vi "MyrioProject.vi"() -> ()   [LabVIEW 2018]
doc: "The myRIO Project template acquires acceleration data from the onboard accelerometer and displays the changes of acceleration values in a waveform chart."
uses:
  <vilib>/myRIO/Common/Instrument Driver Framework/myRIO v1.0/Encoder/typedefs/Encoder Signal Mode.ctl
  <vilib>/Platform/TimedLoop/XDataNode/timing_clust.ctl
  <vilib>/Platform/TimedLoop/XDataNode/nitl_modes.ctl
  <vilib>/Platform/TimedLoop/XDataNode/wakeup.ctl
  <vilib>/Analysis/Matrix/Datatypes/RealMatrix.ctl
  <vilib>/myRIO/Instrument Drivers/Onboard IO/PWM/typedefs/PWM Reference.ctl
  <vilib>/myRIO/Common/Instrument Driver Framework/Utilities/typedefs/myRIO Generic Hardware Reference.ctl
  <vilib>/myRIO/Common/Instrument Driver Framework/Utilities/typedefs/Hardware Version Enum.ctl
  <vilib>/myRIO/Common/Instrument Driver Framework/Utilities/typedefs/myRIO v1.0 Reference.ctl
  <vilib>/myRIO/Common/Instrument Driver Framework/Utilities/typedefs/Generic FPGA Reference.ctl
  <vilib>/myRIO/Common/Instrument Driver Framework/myRIO v1.0/PWM/typedefs/PWM Channels Enum.ctl
  <vilib>/myRIO/Instrument Drivers/Onboard IO/PWM/typedefs/PWM Configuration.ctl
  <vilib>/userdefined/High Color/nirio_resource_hc.ctl
  <vilib>/myRIO/Common/Instrument Driver Framework/myRIO v1.0/Encoder/typedefs/Encoder Configuration v1.0.ctl
  <vilib>/myRIO/Instrument Drivers/Onboard IO/Encoder/typedefs/Encoder Reference.ctl
  <vilib>/myRIO/Common/Instrument Driver Framework/myRIO v1.0/Encoder/typedefs/Encoder Channels Enum.ctl
  <vilib>/myRIO/Instrument Drivers/Onboard IO/DIO/typedefs/DIO Reference.ctl
  <vilib>/myRIO/Common/Instrument Driver Framework/myRIO v1.0/DIO/typedefs/DIO Channels List.ctl
  <vilib>/myRIO/Common/Instrument Driver Framework/myRIO v1.0/DIO/typedefs/DIO Channels Enum.ctl
  <vilib>/myRIO/Instrument Drivers/Onboard IO/AI/typedefs/AI Reference.ctl
  <vilib>/myRIO/Common/Instrument Driver Framework/myRIO v1.0/AI/typedefs/AI Channels List.ctl
  <vilib>/myRIO/Common/Instrument Driver Framework/myRIO v1.0/AI/typedefs/AI Channels Enum.ctl
  <vilib>/myRIO/Common/Instrument Driver Framework/Utilities/typedefs/Analog Scaling Constants List.ctl
  <vilib>/myRIO/Common/Instrument Driver Framework/Utilities/typedefs/Analog Scaling Constants.ctl
  <vilib>/myRIO/Common/Instrument Driver Framework/myRIO v1.0/PWM/vis/myRIO v1.1 Open PWM.vi
  <vilib>/myRIO/Common/Instrument Driver Framework/myRIO v1.0/Encoder/vis/myRIO v1.1 Open Encoder.vi
  <vilib>/myRIO/Common/Instrument Driver Framework/Utilities/vis/Is FPGA Ref Available.vi
  <vilib>/myRIO/Common/Instrument Driver Framework/myRIO v1.0/AI/vis/myRIO v1.1 Open AI.vi
  <vilib>/myRIO/Common/Instrument Driver Framework/myRIO v1.0/DIO/vis/myRIO v1.1 Open DIO.vi
  <vilib>/myRIO/Instrument Drivers/Onboard IO/PWM/vis/Set Duty Cycle and Frequency.vi
  <vilib>/myRIO/Instrument Drivers/Onboard IO/DIO/vis/Write.vi
  <vilib>/myRIO/Common/Instrument Driver Framework/Utilities/vis/Validate Channels.vi
  <vilib>/myRIO/Common/Instrument Driver Framework/myRIO v1.0/PWM/vis/myRIO v1.0 Reserve PWM.vi
  <vilib>/myRIO/Common/Instrument Driver Framework/myRIO v1.0/Encoder/vis/myRIO v1.0 Reserve Encoder.vi
  <vilib>/myRIO/Common/Instrument Driver Framework/myRIO v1.0/AI/vis/myRIO v1.0 Reserve AI.vi
  <vilib>/myRIO/Common/Instrument Driver Framework/myRIO v1.0/DIO/vis/myRIO v1.0 Reserve DIO.vi
  <vilib>/myRIO/Common/Instrument Driver Framework/myRIO v1.0/Encoder/vis/myRIO v1.0 Close Encoder.vi
  <vilib>/myRIO/Common/Instrument Driver Framework/myRIO v1.0/PWM/vis/myRIO v1.0 Close PWM.vi
  <vilib>/myRIO/Common/Instrument Driver Framework/myRIO v1.0/PWM/vis/myRIO v1.0 Build MUX Configuration PWM.vi
  <vilib>/myRIO/Common/Instrument Driver Framework/myRIO v1.0/Resource Manager/vis/myRIO v1.0 Reserve Channel List.vi
  <vilib>/myRIO/Common/Instrument Driver Framework/myRIO v1.0/Encoder/vis/myRIO v1.0 Build MUX Configuration Encoder.vi
  <vilib>/myRIO/Common/Instrument Driver Framework/myRIO v1.0/AI/vis/myRIO v1.0 Build MUX Configuration AI.vi
  <vilib>/myRIO/Common/Instrument Driver Framework/myRIO v1.0/DIO/vis/myRIO v1.0 Build MUX Configuration DIO.vi
  <vilib>/myRIO/Common/Instrument Driver Framework/myRIO v1.0/Encoder/vis/myRIO v1.0 Unreserve Encoder.vi
  <vilib>/myRIO/Common/Instrument Driver Framework/myRIO v1.0/PWM/vis/myRIO v1.0 Unreserve PWM.vi
  <vilib>/myRIO/Common/Instrument Driver Framework/myRIO v1.0/Resource Manager/vis/myRIO v1.0 Create Configuration List.vi
  <vilib>/myRIO/Common/Instrument Driver Framework/myRIO v1.0/Resource Manager/vis/myRIO v1.0 Reserve Channel.vi
  <vilib>/myRIO/Common/Instrument Driver Framework/myRIO v1.0/Resource Manager/vis/myRIO v1.0 Unreserve Channel.vi
  <vilib>/myRIO/Common/Instrument Driver Framework/myRIO v1.0/Resource Manager/vis/myRIO v1.0 Unreserve Channel List.vi
  <vilib>/myRIO/Common/Instrument Driver Framework/myRIO v1.0/Resource Manager/vis/myRIO v1.0 Build Mutex Name.vi
  <vilib>/Utility/VariantDataType/GetNumericInfo.vi
  <vilib>/Utility/error.llb/Error Cluster From Error Code.vi
  <vilib>/myRIO/Common/Instrument Driver Framework/myRIO v1.0/myRIO v1.1 Open.vi
  <vilib>/myRIO/Common/Instrument Driver Framework/Utilities/vis/IO Manager.vi
  <vilib>/myRIO/Common/Instrument Driver Framework/Utilities/vis/Configuration Manager.vi
  <vilib>/myRIO/Common/Instrument Driver Framework/myRIO v1.0/Resource Manager/vis/myRIO v1.0 Configure IO.vi
  <vilib>/myRIO/Common/Instrument Driver Framework/myRIO v1.0/myRIO v1.0 Close.vi
  <vilib>/myRIO/Common/Instrument Driver Framework/myRIO v1.0/PWM/vis/myRIO v1.0 Write PWM.vi
  <vilib>/myRIO/Common/Instrument Driver Framework/myRIO v1.0/Encoder/vis/myRIO v1.0 Configure Encoder.vi
  <vilib>/myRIO/Common/Instrument Driver Framework/myRIO v1.0/Encoder/vis/myRIO v1.0 Enable Encoder.vi
  <vilib>/myRIO/Common/Instrument Driver Framework/myRIO v1.0/DIO/vis/myRIO v1.0 Read DIO.vi
  <vilib>/myRIO/Common/Instrument Driver Framework/myRIO v1.0/AI/vis/myRIO v1.0 Get Scaling Constants AI.vi
  <vilib>/myRIO/Common/Instrument Driver Framework/myRIO v1.0/AI/vis/myRIO v1.0 Read AI.vi
  <vilib>/myRIO/Common/Instrument Driver Framework/myRIO v1.0/Encoder/vis/myRIO v1.0 Read Encoder.vi
  <vilib>/myRIO/Common/Instrument Driver Framework/myRIO v1.0/DIO/vis/myRIO v1.0 Write DIO.vi
  <vilib>/myRIO/Common/Instrument Driver Framework/myRIO v1.0/Encoder/vis/myRIO v1.0 Shutdown Encoder.vi
  <vilib>/myRIO/Common/Instrument Driver Framework/myRIO v1.0/PWM/vis/myRIO v1.0 Shutdown PWM.vi
  <vilib>/platform/TimedLoop/XDataNode/XDataNode.xnode
  <vilib>/myRIO/Instrument Drivers/Onboard IO/PWM/vis/myRIO PWM Open.xnode
  <vilib>/myRIO/Instrument Drivers/Onboard IO/Encoder/vis/myRIO Encoder Open.xnode
  <vilib>/myRIO/Express VI/Onboard Devices/Button/Button Express VI.xnode
  <vilib>/myRIO/Instrument Drivers/Onboard IO/DIO/vis/myRIO DIO Open.xnode
  <vilib>/myRIO/Express VI/Onboard IO/AI/AI Express VI.xnode
  <vilib>/myRIO/Instrument Drivers/Onboard IO/AI/vis/myRIO AI Open.xnode
  <vilib>/myRIO/Express VI/Onboard IO/PWM/PWM Express VI.xnode
  <vilib>/myRIO/Express VI/Onboard IO/DO/DO Express VI.xnode
  <vilib>/myRIO/Instrument Drivers/Onboard IO/Encoder/Encoder.lvlib
  <vilib>/myRIO/Instrument Drivers/Onboard IO/PWM/PWM.lvlib
  <vilib>/myRIO/Instrument Drivers/Onboard IO/DIO/DIO.lvlib
  <vilib>/myRIO/Instrument Drivers/Onboard IO/AI/AI.lvlib
  <vilib>/Platform/TimedLoop/XDataNode/XDNodeRunTimeDep.lvlib
  <vilib>/Analysis/Matrix/NI_Matrix.lvlib
panel:
  in  "pequeoffset":dbl
  in  "s":bool
  in  "grandeoffset":dbl
  in  "saturacion 2":dbl=0.3
  in  "Garra":bool
  out "stall":bool
  in  "Start":bool
  in  "Stop Button":bool
  out "element":dbl
  out "element 2":dbl
  in  "manual":bool
  out "data":dbl
  out "sensor2 (A/AI2 (Pin 7))":dbl
  out "sensor1":dbl
  out "stallRojo (A/AI0 (Pin 3))":dbl
  out "stallBlanco (A/AI1 (Pin 5))":dbl
  out "subarray 2":dbl[][](array[numeric])
  out "subarray":dbl[][](array[numeric])
  out "vectores":dbl[][][](array[numeric])
  in  "saturacion":dbl=0.3
  in  "Garra":dbl(slide)=0.5 scale=0.05..0.1
  in  "Subir":dbl(slide)=0.5 scale=0.05..0.15
  in  "Reset Counter 2":bool
  in  "Reset Counter":bool
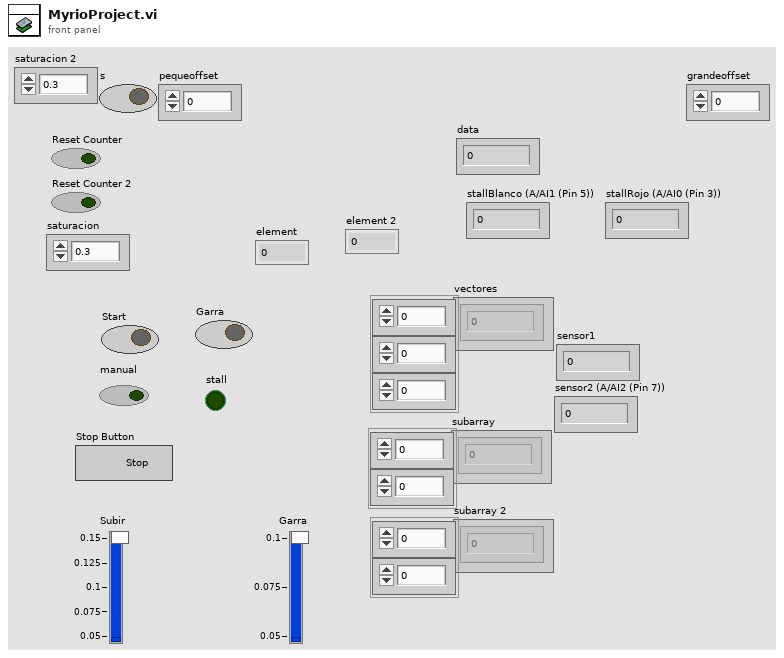
[diagram p1: front panel]
types:
  T1 = enum16{"Up-Closed", "Baja-abre", "cierra", "sube"}
  T2 = typedef "NI_Matrix.lvlib/RealMatrix.ctl" = dbl[][]
  T3 = enum16{"normal", "grande-Sensor", "grande home", "peque-sensor", "peque- home", "peque-reset"}
  T4 = typedef "Encoder Signal Mode.ctl" = enum16{"Quadrature phase signal", "Step and direction signal"}
  T5 = typedef "PWM.lvlib/PWM Reference.ctl" = cluster{"myRIO Reference":T6, "PWM Channels Enum":T10, "PWM Configuration":T11}
  T6 = typedef "myRIO Generic Hardware Reference.ctl" = cluster{"myRIO Model":T7, "myRIO Hardware Reference":T8}
  T7 = typedef "Hardware Version Enum.ctl" = enum16{"Unknown", "myRIO-1900", "myRIO-1950", "roboRIO", "NI ELVIS RIO CM", "ELVIS III"}
  T8 = typedef "myRIO v1.0 Reference.ctl" = cluster{"Generic FPGA Reference":T9, "Allow multiple opens":bool}
  T9 = typedef "Generic FPGA Reference.ctl" = refnum<k20>
  T10 = typedef "PWM Channels Enum.ctl" = enum16{"Not Connected", "C/PWM0", "C/PWM1", "A/PWM0", "A/PWM1", "A/PWM2", "A/PWM3", "A/PWM4", "A/PWM5", "A/PWM6", "A/PWM7", "A/PWM8", "A/PWM9", "A/PWM10", "A/PWM11", "A/PWM12", "A/PWM13", "A/PWM14", "A/PWM15", "A/PWM16", "A/PWM17", "A/PWM18", "A/PWM19", "B/PWM0", "B/PWM1", "B/PWM2", "B/PWM3", "B/PWM4", "B/PWM5", "B/PWM6", "B/PWM7", "B/PWM8", "B/PWM9", "B/PWM10", "B/PWM11", "B/PWM12", "B/PWM13", "B/PWM14", "B/PWM15", "B/PWM16", "B/PWM17", "B/PWM18", "B/PWM19", "PWM/PWM0", "PWM/PWM1", "PWM/PWM2", "PWM/PWM3", "PWM/PWM4", "PWM/PWM5", "PWM/PWM6", "PWM/PWM7", "PWM/PWM8", "PWM/PWM9"}
  T11 = typedef "PWM.lvlib/PWM Configuration.ctl" = cluster{"Frequency":dbl, "Duty Cycle":dbl}
  T12 = typedef "Encoder.lvlib/Encoder Reference.ctl" = cluster{"myRIO Reference":T6, "Encoder Channels Enum":T13}
  T13 = typedef "Encoder Channels Enum.ctl" = enum16{"Not Connected", "C/ENC0", "C/ENC1", "A/ENC", "A/ENC0", "A/ENC1", "A/ENC2", "A/ENC3", "A/ENC4", "A/ENC5", "A/ENC6", "A/ENC7", "A/ENC8", "A/ENC9", "B/ENC", "B/ENC0", "B/ENC1", "B/ENC2", "B/ENC3", "B/ENC4", "B/ENC5", "B/ENC6", "B/ENC7", "B/ENC8", "B/ENC9", "DIO/ENC0", "DIO/ENC1", "DIO/ENC2", "DIO/ENC3", "DIO/ENC4"}
  T14 = cluster{"Double":dbl, "dbl Scaled Value":dbl, "Output":dbl, "seconds since 1Jan1904":timestamp, dbl, dbl, dbl}
  T15 = typedef "XDNodeRunTimeDep.lvlib/timing_clust.ctl" = cluster{"Expected End [f-1]":u64, "Actual End [f-1]":u64, "Finished Late? [f-1]":bool, "Expected End [i-1]":u64, "Actual End [i-1]":u64, "Finished Late? [i-1]":bool, "Expected Start [i]":u64, "Actual Start [i]":u64, "Expected Start [f]":u64, "Actual Start [f]":u64, "Source Name":string, "Structure Name":string, "Period":i64, "Deadline":i64, "Offset":i64, "Start":i64, "Priority":i32, "Timeout":i32, "Mode":T16, "Wakeup Reason":T17, "Error":errorcluster, "Source Type":string, "Secondary Source Type":string, "Global End Time":u64, "Global Start Time":u64, "Frame Duration":u64, "Iteration Duration":u64, "Assigned CPU":i32, "I/O Scan Engine Mode":u32}
  T16 = typedef "XDNodeRunTimeDep.lvlib/nitl_modes.ctl" = enum32{"No Change", "Process missed periods, maintain original phase", "Discard missed periods, maintain original phase", "Process missed periods, ignore original phase", "Discard missed periods, ignore original phase"}
  T17 = typedef "XDNodeRunTimeDep.lvlib/wakeup.ctl" = enum32{"Normal", "Aborted", "Asynchronous wakeup", "Timing source error", "Timed loop error", "Timeout"}
  T18 = typedef "nirio_resource_hc.ctl" = tag
  T19 = typedef "AI.lvlib/AI Reference.ctl" = cluster{"myRIO Reference":T6, "AI Channels List":T20, "AI Scaling Constants List":T22}
  T20 = typedef "AI Channels List.ctl" = T21[]
  T21 = typedef "AI Channels Enum.ctl" = enum16{"Not Connected", "AudioIn/Left", "AudioIn/Right", "C/AI0", "C/AI1", "A/AI0", "A/AI1", "A/AI2", "A/AI3", "A/AI4", "A/AI5", "A/AI6", "A/AI7", "B/AI0", "B/AI1", "B/AI2", "B/AI3", "B/AI4", "B/AI5", "B/AI6", "B/AI7", "AI/AI0", "AI/AI1", "AI/AI2", "AI/AI3", "A/AI0 (DIFF)", "A/AI1 (DIFF)", "A/AI2 (DIFF)", "A/AI3 (DIFF)", "B/AI0 (DIFF)", "B/AI1 (DIFF)", "B/AI2 (DIFF)", "B/AI3 (DIFF)"}
  T22 = typedef "Analog Scaling Constants List.ctl" = T23[]
  T23 = typedef "Analog Scaling Constants.ctl" = cluster{"LSB Weight (Volts)":dbl, "Offset (Volts)":dbl, "Signed?":bool}
  T24 = typedef "DIO.lvlib/DIO Reference.ctl" = cluster{"myRIO Reference":T6, "DIO Channels List":T25}
  T25 = typedef "DIO Channels List.ctl" = T26[]
  T26 = typedef "DIO Channels Enum.ctl" = enum16{"Not Connected", "C/DIO0", "C/DIO1", "C/DIO2", "C/DIO3", "C/DIO4", "C/DIO5", "C/DIO6", "C/DIO7", "A/DIO0", "A/DIO1", "A/DIO2", "A/DIO3", "A/DIO4", "A/DIO5", "A/DIO6", "A/DIO7", "A/DIO8", "A/DIO9", "A/DIO10", "A/DIO11", "A/DIO12", "A/DIO13", "A/DIO14", "A/DIO15", "A/DIO16", "A/DIO17", "A/DIO18", "A/DIO19", "B/DIO0", "B/DIO1", "B/DIO2", "B/DIO3", "B/DIO4", "B/DIO5", "B/DIO6", "B/DIO7", "B/DIO8", "B/DIO9", "B/DIO10", "B/DIO11", "B/DIO12", "B/DIO13", "B/DIO14", "B/DIO15", "B/DIO16", "B/DIO17", "B/DIO18", "B/DIO19", "LED0", "LED1", "LED2", "LED3", "Button0", "DIO/DIO0", "DIO/DIO1", "DIO/DIO2", "DIO/DIO3", "DIO/DIO4", "DIO/DIO5", "DIO/DIO6", "DIO/DIO7", "DIO/DIO8", "DIO/DIO9", "SPI/CS0", "SPI/CS1", "SPI/CS2", "SPI/CS3", "LED RADIO (Green)", "LED RADIO (Red)", "LED COMM (Green)", "LED COMM (Red)", "LED MODE (Green)", "LED MODE (Red)"}
  T27 = cluster{dbl, "Perturbacion":dbl, dbl, "seconds since 1Jan1904":timestamp, dbl, dbl, dbl}
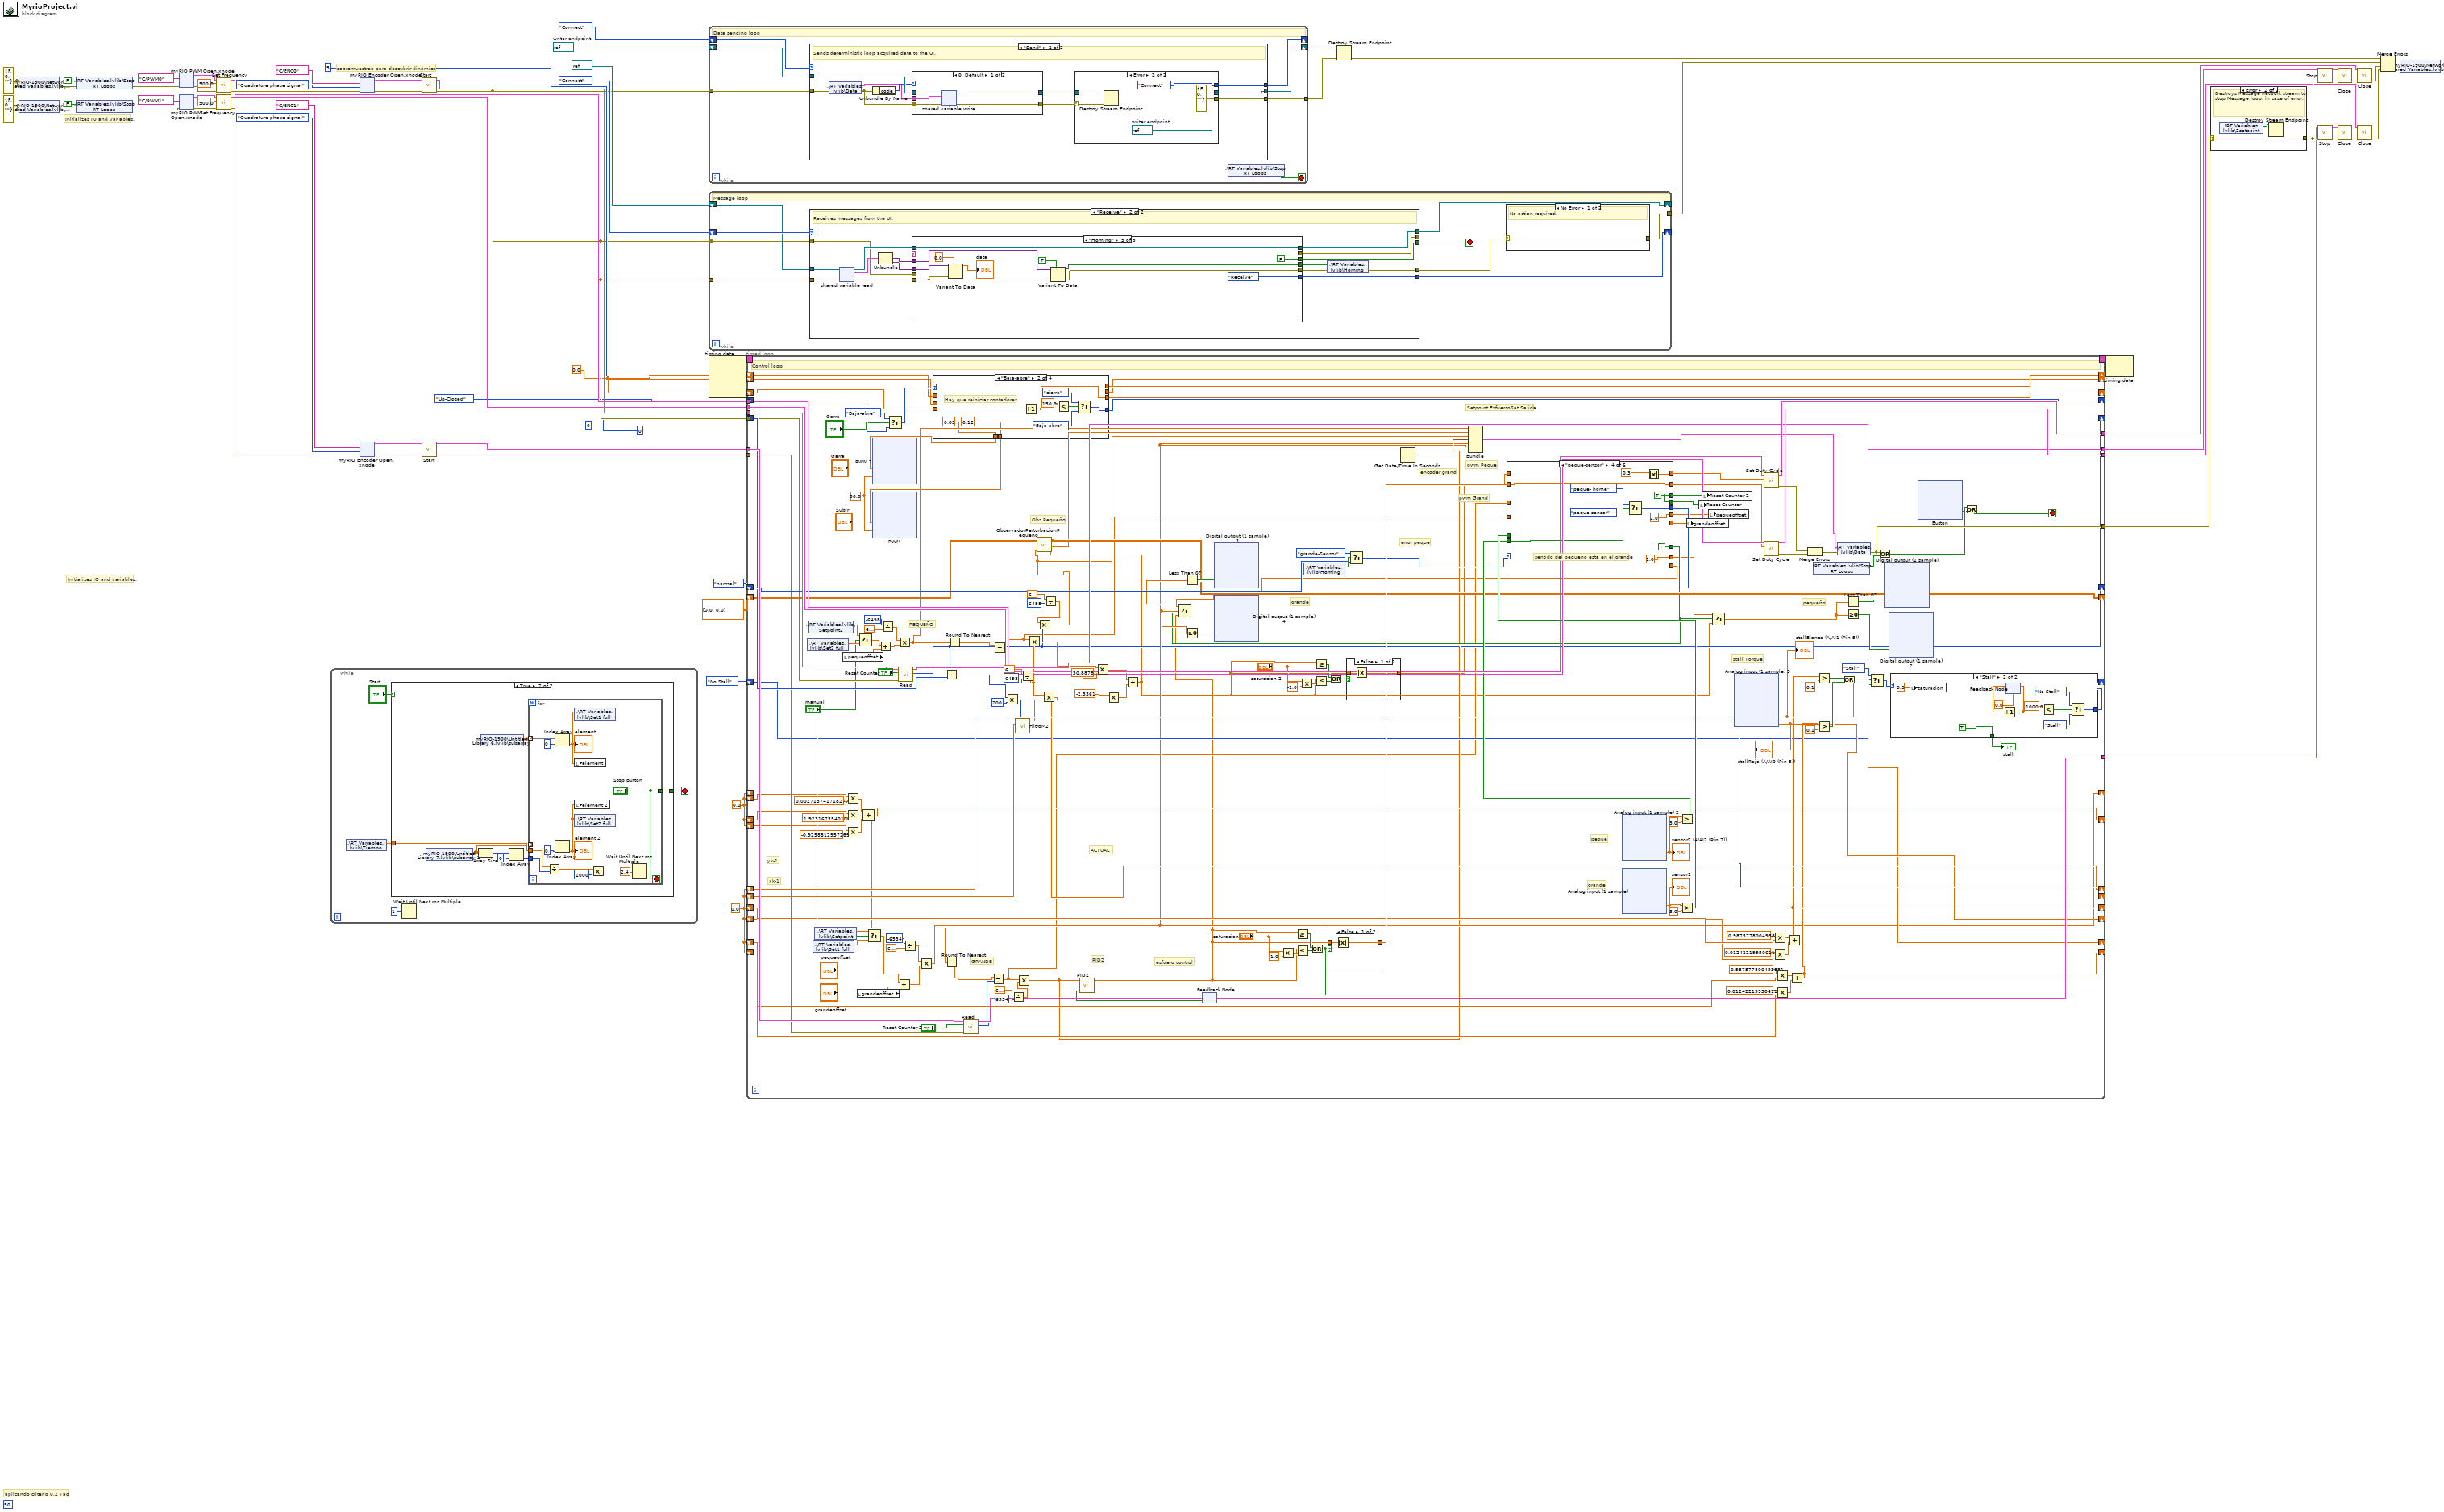
[diagram p0: block diagram]
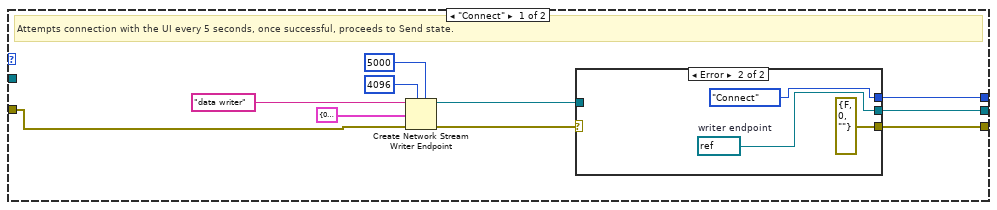
[diagram p4: hidden frame]
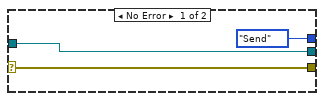
[diagram p5: hidden frame]
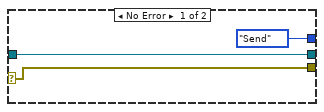
[diagram p6: hidden frame]
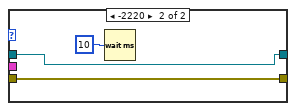
[diagram p7: hidden frame]
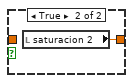
[diagram p8: hidden frame]
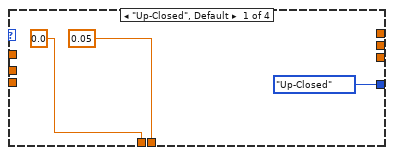
[diagram p9: hidden frame]
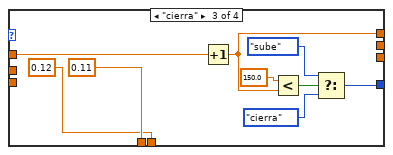
[diagram p10: hidden frame]
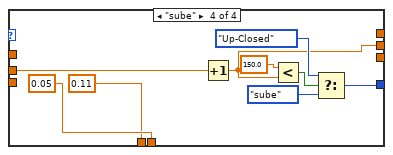
[diagram p11: hidden frame]
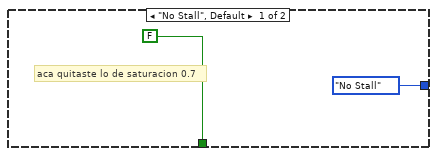
[diagram p12: hidden frame]
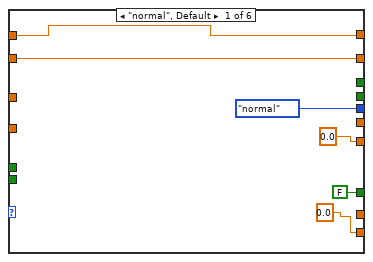
[diagram p13: hidden frame]
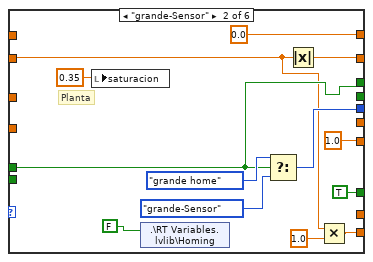
[diagram p14: hidden frame]
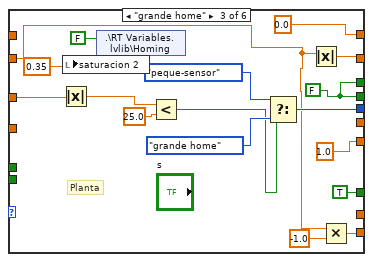
[diagram p15: hidden frame]
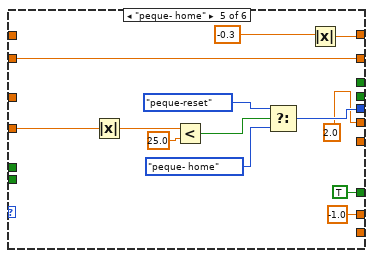
[diagram p16: hidden frame]
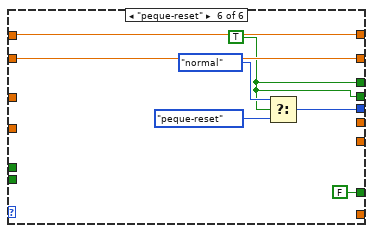
[diagram p17: hidden frame]
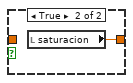
[diagram p18: hidden frame]
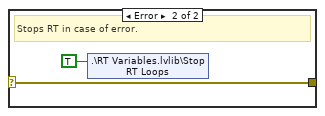
[diagram p19: hidden frame]
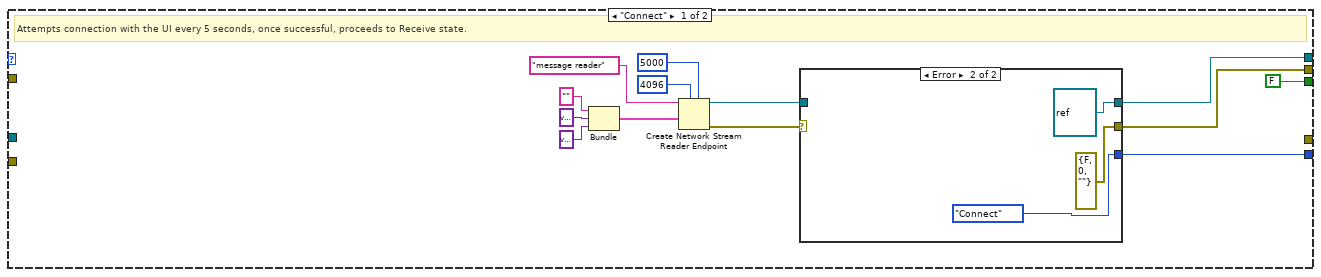
[diagram p20: hidden frame]
diagram:
  w1 = 0.0
  w2 = 0.0
  w5 = 0.0
  (unwired) 0
  (unwired) 50
  w20 = refnum<k21> refnum  # writer endpoint
  w33 = errorcluster {"status"=FALSE, "code"=0, "source"=""} ("error IO")
  w55 = errorcluster {"status"=FALSE, "code"=0, "source"=""} ("error IO")
  # "aplicando criterio 0.2 Tao"
  # "sobremuestreo para descubrir dinámica"
  # "Initializes IO and variables."
  # "Initializes IO and variables."
  n1 = shared-variable "myRIO-1900\\Network Shared Variables.lvlib\\error IO"(w55, error in=w55) -> (error out=w56:errorcluster)
  n2 = shared-variable "myRIO-1900\\Network Shared Variables.lvlib\\error IO"(w33, error in=w33) -> (error out=w34:errorcluster)
  n3 = shared-variable ".\\RT Variables.lvlib\\Stop RT Loops"(FALSE ("Stop RT Loops"), error in=w56) -> (error out=w43:errorcluster)
  n4 = shared-variable ".\\RT Variables.lvlib\\Stop RT Loops"(FALSE ("Stop RT Loops"), error in=w34) -> (error out=w26:errorcluster)
  n5 = xnode "myRIO PWM Open.xnode"("error in (no error)"=w43, "Channel Name"=tag "C/PWM0") -> ("error out"=w45:errorcluster, "PWM Ref Out"=w44:T5)  [unwired: 1 in]
  n6 = xnode "myRIO PWM Open.xnode"("error in (no error)"=w26, "Channel Name"=tag "C/PWM1") -> ("error out"=w28:errorcluster, "PWM Ref Out"=w27:T5)  [unwired: 1 in]
  n7 = call <vilib>:"Set Frequency.vi"("error in (no error)"=w45, "Frequency [Hz]"=500.0, "PWM Ref In"=w44) -> ("error out"=w42:errorcluster, "PWM Ref Out"=w39:T5)  [unwired: 6 in]
  n8 = call <vilib>:"Set Frequency.vi"("error in (no error)"=w28, "Frequency [Hz]"=500.0, "PWM Ref In"=w27) -> ("error out"=w25:errorcluster, "PWM Ref Out"=w21:T5)  [unwired: 6 in]
  n9 = while {
    stop <- w67 stop-if-true
    n10 = shared-variable ".\\RT Variables.lvlib\\Tiempo"() -> (w69:dbl)  [unwired: 1 in, 1 out]
    n11 = case shown="True" "Start" {
      tunnel: w69 -> [_ w76]
      tunnel: [_ w75] -> w67
      frame False {
      }
      frame True {
        n12 = shared-variable "myRIO-1900\\Untitled Library 7.lvlib\\subarray 2"() -> (w74:dbl[][])  [unwired: 1 in, 1 out]
        n13 = Array Size(array=w74) -> (size(s)=w72:i32[])
        n14 = shared-variable "myRIO-1900\\Untitled Library 6.lvlib\\subarray"() -> (w77:dbl[][])  [unwired: 1 in, 1 out]
        n15 = Index Array(array=w72, index=0) -> (element=w71:i32)
        n16 = for {
          tunnel: w77 -> [w87] mode=indexing
          tunnel: w74 -> [w84] mode=indexing
          tunnel: w76 -> [w81]
          tunnel: ["Stop Button"] -> w75
          tunnel: w71 -> [w79]
          stop <- "Stop Button" stop-if-true
          n17 = Divide(x=w81, y=w79) -> (x/y=w89:dbl)
          n18 = Index Array(array=w87, index=0) -> (element=w83:dbl)
          "element" <- w83
          n19 = Index Array(array=w84, index=0) -> (element=w82:dbl)
          "element 2" <- w82
          n20 = shared-variable ".\\RT Variables.lvlib\\Set1 full"(w83) -> ()  [unwired: 1 in, 1 out]
          n21 = local write "element"(w83) -> ()
          n22 = local write "element 2"(w82) -> ()
          n23 = shared-variable ".\\RT Variables.lvlib\\Set2 full"(w82) -> ()  [unwired: 1 in, 1 out]
          n24 = Multiply(x=w89, y=1000) -> ()  [unwired: 1 out]
          n25 = Wait Until Next ms Multiple(millisecond multiple=2.4) -> ()  [unwired: 1 out]
        }
      }
    }
    n26 = Wait Until Next ms Multiple(millisecond multiple=u32 1) -> ()  [unwired: 1 out]
  }
  n27 = xnode "myRIO Encoder Open.xnode"("error in (no error)"=w42, "Channel Name"=tag "C/ENC0", "Encoder Signal Mode"=Encoder_Signal_Mode."Quadrature phase signal") -> ("error out"=w52:errorcluster, "Encoder Ref Out"=w51:T12)  [unwired: 2 in]
  n28 = xnode "myRIO Encoder Open.xnode"("error in (no error)"=w25, "Channel Name"=tag "C/ENC1", "Encoder Signal Mode"=Encoder_Signal_Mode."Quadrature phase signal") -> ("error out"=w31:errorcluster, "Encoder Ref Out"=w30:T12)  [unwired: 2 in]
  n29 = call <vilib>:"Start.vi"("error in (no error)"=w52, "Encoder Ref In"=w51) -> ("error out"=w10:errorcluster, "Encoder Ref Out"=w49:T12)  [unwired: 8 in]
  n30 = call <vilib>:"Start.vi"("error in (no error)"=w31, "Encoder Ref In"=w30) -> ("error out"=w9:errorcluster, "Encoder Ref Out"=w22:T12)  [unwired: 8 in]
  n31 = while {
    shift-right: [w94] -> w61
    shift-left: w20 -> [w92]
    tunnel: [w93] -> w62
    tunnel: w10 -> [w91]
    shift-right: [w90] -> _
    shift-left: enum16{"Connect", "Send"}."Connect" ("Message states") -> [w95]
    stop <- w96 stop-if-true
    # "Data sending loop"
    n32 = case shown="\"Send\"" w95 {
      tunnel: [w100 w115] -> w93
      tunnel: [w98 w113] -> w94
      tunnel: [w104 w116] -> w90
      tunnel: w92 -> [_ w122]
      tunnel: w91 -> [w101 w121]
      frame "Connect" {
        # "Attempts connection with the UI every 5 seconds, once successful, proceeds to Send state."
        n33 = Create Network Stream Writer Endpoint(5:5000 ("timeout in ms (-1)"), 7:4096 ("writer buffer size"), 8:w101, 9:T14 {"Double"=0.0, "dbl Scaled Value"=0.0, "Output"=0.0, "seconds since 1Jan1904"=timestamp(0 s since 1904-01-01), 0.0, 0.0, 0.0} ("Data"), 11:"data writer" ("writer name")) -> (0:w102:errorcluster, 3:w99:refnum<k21>)  [unwired: 2 in]
        n34 = case shown="Error" w102 {
          selector: w102 -> [w107 _]
          tunnel: [enum16{"Connect", "Send"}."Send" ("Message states") enum16{"Connect", "Send"}."Connect" ("Message states")] -> w104
          tunnel: [w107 errorcluster {"status"=FALSE, "code"=0, "source"=""} ("error IO")] -> w100
          tunnel: w99 -> [w109 _]
          tunnel: [w109 w110] -> w98
          frame No Error {
          }
          frame Error {
            w110 = refnum<k21> refnum  # writer endpoint
          }
        }
      }
      frame "Send" {
        # "Sends deterministic loop acquired data to the UI."
        n35 = shared-variable ".\\RT Variables.lvlib\\Data"(error in=w121) -> (w118:T14, error out=w120:errorcluster)
        n36 = Unbundle By Name(w120) -> ("code"=w119:i32)
        n37 = case shown="0, Default" w119 {
          tunnel: [w135 w137] -> w117
          tunnel: [w134 w136] -> w114
          tunnel: w122 -> [w133 w136]
          tunnel: w120 -> [w132 w137]
          tunnel: w118 -> [w131 _]
          frame 0, Default {
            n38 = shared-variable-write(w133, w132, w131) -> (w134:refnum<k21>, w135:errorcluster)  [unwired: 1 in, 1 out]
          }
          frame -2220 {
            n39 = Wait (ms)(milliseconds to wait=u32 10) -> ()  [unwired: 1 out]
          }
        }
        n40 = case shown="Error" w117 {
          selector: w117 -> [w125 w129]
          tunnel: [enum16{"Connect", "Send"}."Send" ("Message states") enum16{"Connect", "Send"}."Connect" ("Message states")] -> w116
          tunnel: [w125 errorcluster {"status"=FALSE, "code"=0, "source"=""} ("error IO")] -> w115
          tunnel: w114 -> [w123 w128]
          tunnel: [w123 w126] -> w113
          frame No Error {
          }
          frame Error {
            w126 = refnum<k21> refnum  # writer endpoint
            n41 = Destroy Stream Endpoint(8:w129, 11:w128) -> ()  [unwired: 1 out]
          }
        }
      }
    }
    n42 = shared-variable ".\\RT Variables.lvlib\\Stop RT Loops"() -> (w96:bool)  [unwired: 1 in, 1 out]
  }
  n43 = while {
    tunnel: [w142] -> w58
    shift-right: [w146] -> _
    shift-left: refnum<k21> refnum ("reader endpoint") -> [w144]
    shift-right: [w145] -> _
    shift-left: enum16{"Connect", "Receive"}."Connect" ("Message states") -> [w147]
    tunnel: w10 -> [w143]
    tunnel: w10 -> [w140]
    stop <- w141 stop-if-true
    # "Message loop"
    n44 = case shown="\"Receive\"" w147 {
      tunnel: [w154 w171] -> _
      tunnel: [w152 w183] -> w146
      tunnel: [w161 w180] -> w145
      tunnel: w144 -> [_ w179]
      tunnel: w143 -> [_ w182]
      tunnel: [FALSE ("Stop RT Loops") w181] -> w141
      tunnel: w140 -> [_ w176]
      tunnel: [_ w172] -> w139
      frame "Connect" {
        # "Attempts connection with the UI every 5 seconds, once successful, proceeds to Receive state."
        n45 = Bundle("", variant, variant) -> (w157:cluster{string, variant, variant})  [unwired: 1 in]
        n46 = Create Network Stream Reader Endpoint(5:5000 ("timeout in ms (-1)"), 7:4096 ("reader buffer size"), 9:w157, 11:"message reader" ("reader name")) -> (0:w156:errorcluster, 3:w151:refnum<k21>)  [unwired: 3 in]
        n47 = case shown="Error" w156 {
          selector: w156 -> [w166 _]
          tunnel: [enum16{"Connect", "Receive"}."Receive" ("Message states") enum16{"Connect", "Receive"}."Connect" ("Message states")] -> w161
          tunnel: [w165 errorcluster {"status"=FALSE, "code"=0, "source"=""} ("error IO")] -> w154
          tunnel: [w164 refnum<k21> refnum ("reader endpoint")] -> w152
          tunnel: w151 -> [w164 _]
          frame No Error {
            n48 = shared-variable ".\\RT Variables.lvlib\\2setpoint"(w164, error in=w166) -> (error out=w165:errorcluster)
          }
          frame Error {
          }
        }
      }
      frame "Receive" {
        # "Receives messages from the UI."
        n49 = shared-variable-read(w179, w182) -> (w178:refnum<k21>, w184:errorcluster, w175:cluster{string, variant, variant})  [unwired: 1 in, 1 out]
        n50 = Unbundle(w175) -> (w186:string, w185:variant, w177:variant)
        n51 = case shown="\"Homing\"" w186 {
          tunnel: w185 -> [_ w207 w222 w228 w246]
          tunnel: w184 -> [w191 w209 w211 w227 w240]
          tunnel: [w190 w204 w218 w229 _] -> w171
          tunnel: [refnum<k21> refnum ("reader endpoint") refnum<k21> refnum ("reader endpoint") w217 w235 w244] -> w183
          tunnel: w178 -> [w189 w203 w217 w235 w244]
          tunnel: [w187 w206 FALSE ("Stop RT Loops") FALSE ("Stop RT Loops") FALSE ("Stop RT Loops")] -> w181
          tunnel: [enum16{"Connect", "Receive"}."Connect" ("Message states") enum16{"Connect", "Receive"}."Receive" ("Message states") enum16{"Connect", "Receive"}."Receive" ("Message states") enum16{"Connect", "Receive"}."Receive" ("Message states") enum16{"Connect", "Receive"}."Receive" ("Message states")] -> w180
          tunnel: w177 -> [_ w199 w210 w231 w239]
          tunnel: w176 -> [_ w198 _ _ _]
          tunnel: [w187 _ _ _ w237] -> w174
          tunnel: [_ _ _ _ w236] -> w173
          frame "Disconnect UI", Default {
            w187 = FALSE ("Stop RT Loops")
            n52 = Destroy Stream Endpoint(8:w191, 11:w189) -> (0:w190:errorcluster)
          }
          frame "Stop" {
            n53 = Variant To Data(error in=w209, type=TRUE ("Stop RT Loops"), Variant=w207) -> (data=w206:bool, error out=w208:errorcluster)
            n54 = Variant To Data(error in=w198, type=TRUE ("Stop RT Loops"), Variant=w199) -> (data=w196:bool, error out=w200:errorcluster)
            n55 = shared-variable ".\\RT Variables.lvlib\\Stop RT Loops"(w206, error in=w208) -> (error out=w194:errorcluster)
            n56 = shared-variable ".\\RT Variables.lvlib\\Stop RT Loops"(w196, error in=w200) -> (error out=w195:errorcluster)
            n57 = Merge Errors(w194, w195) -> (w193:errorcluster)
            n58 = Destroy Stream Endpoint(8:w193, 11:w203) -> (0:w204:errorcluster)
          }
          frame "Update setpoint" {
            n59 = Variant To Data(error in=w211, type=0.0, Variant=w222) -> (data=w220:dbl, error out=w219:errorcluster)
            n60 = Variant To Data(error in=w211, type=0.0, Variant=w210) -> (data=w213:dbl, error out=w212:errorcluster)
            n61 = shared-variable ".\\RT Variables.lvlib\\Setpoint2"(w213, error in=w212) -> ()  [unwired: 1 out]
            n62 = shared-variable ".\\RT Variables.lvlib\\Setpoint"(w220, error in=w219) -> (error out=w218:errorcluster)
          }
          frame "Vector Setpoints" {
            n63 = Variant To Data(error in=w227, type=0.0, Variant=w231) -> (data=w230:dbl)  [unwired: 1 out]
            n64 = Variant To Data(error in=w227, type=dbl[][][] [], Variant=w228) -> (data=w225:dbl[][][])  [unwired: 1 out]
            "vectores" <- w225
            n65 = Index Array(array=w225) -> (element #1=w224:dbl[][], element #2=w223:dbl[][])  [unwired: 6 in]
            "subarray" <- w224
            "subarray 2" <- w223
            n66 = shared-variable "myRIO-1900\\Untitled Library 6.lvlib\\subarray"(w224) -> ()  [unwired: 1 in, 1 out]
            n67 = shared-variable "myRIO-1900\\Untitled Library 7.lvlib\\subarray 2"(w223) -> ()  [unwired: 1 in, 1 out]
            n68 = shared-variable ".\\RT Variables.lvlib\\Tiempo"(w230) -> (error out=w229:errorcluster)  [unwired: 1 in]
          }
          frame "Homing" {
            n69 = Variant To Data(error in=w240, type=0.0, Variant=w239) -> (data=→"data":dbl)  [unwired: 1 out]
            n70 = Variant To Data(error in=w240, type=TRUE, Variant=w246) -> (data=w237:bool, error out=w236:errorcluster)
          }
        }
        n71 = shared-variable ".\\RT Variables.lvlib\\Homing"(w174, error in=w173) -> (error out=w172:errorcluster)
      }
    }
    n72 = case shown="No Error" w139 {
      selector: w139 -> [w148 w149]
      tunnel: [w148 w149] -> w142
      frame No Error {
        # "No action required."
      }
      frame Error {
        # "Stops RT in case of error."
        n73 = shared-variable ".\\RT Variables.lvlib\\Stop RT Loops"(TRUE ("Stop RT Loops")) -> ()  [unwired: 1 in, 1 out]
      }
    }
  }
  n74 = node-c288(i64 5 ("Period")) -> (w66:T15)  [unwired: 3 in]
  n75 = timed-loop {
    timing: w66 -> [_]
    timing-out: [_] -> w65
    tunnel: [w411] -> w54
    tunnel: w49 -> [w393]
    tunnel: [w392] -> w46
    tunnel: w39 -> [w383]
    tunnel: [w410] -> w38
    tunnel: w22 -> [w407]
    tunnel: w21 -> [w406]
    tunnel: [w402] -> w15
    tunnel: [w401] -> w14
    shift-right: [w382] -> _
    shift-left: T3."normal" ("Enum") -> [w381]
    shift-right: [w268] -> _
    shift-left: 0 -> [w371]
    tunnel: w9 -> [w369]
    tunnel: w10 -> [w368]
    shift-right: [w343] -> _
    shift-left: w5 -> [w342]
    shift-right: [w339] -> _
    shift-left: w5 -> [w341]
    shift-right: [w335] -> _
    shift-left: T2 [[0.0], [0.0]] ("A + B") -> [w334]
    shift-right: [w314] -> _
    shift-left: w5 -> [w324]
    shift-right: [w313] -> _
    shift-left: w5 -> [w319]
    shift-right: [w318] -> _
    shift-left: w5 -> [w317]
    shift-right: [w316] -> _
    shift-left: w5 -> [w315]
    shift-right: [w304] -> _
    shift-left: enum16{"No Stall", "Stall"}."No Stall" -> [w303]
    shift-right: [w298] -> _
    shift-left: T1."Up-Closed" -> [w297]
    shift-right: [w294] -> _
    shift-left: w2 -> [w295]
    shift-right: [w290] -> _
    shift-left: w2 -> [w293]
    shift-right: [w291] -> _
    shift-left: w2 -> [w292]
    shift-right: [w274] -> _
    shift-left: w1 -> [_]
    shift-right: [w272] -> _
    shift-left: w1 -> [w280]
    shift-left: w1 -> [w281]
    shift-left: w1 -> [w279]
    stop <- w399 stop-if-true
    w370 = 50.0 ("Frequency [Hz]")
    # "grande"
    # "pequeño"
    # "ACTUAL"
    # "PID2"
    # "error peque"
    # "encoder grand"
    # "pwm Grand"
    # "pwm Peque"
    # "esfuero control"
    # "Obs Pequeño"
    # "yk-1"
    # "xk-1"
    # "PEQUEÑO"
    # "peque"
    # "grande"
    # "stall Torque"
    # "Setpoint,EsfuersoSat,Salida"
    # "GRANDE"
    # "Control loop"
    n76 = shared-variable ".\\RT Variables.lvlib\\Set2 full"() -> (w332:dbl)  [unwired: 1 in, 1 out]
    n77 = shared-variable ".\\RT Variables.lvlib\\Setpoint2"() -> (w333:dbl)  [unwired: 1 in, 1 out]
    n78 = shared-variable ".\\RT Variables.lvlib\\Set1 full"() -> (w330:dbl)  [unwired: 1 in, 1 out]
    n79 = shared-variable ".\\RT Variables.lvlib\\Setpoint"() -> (w331:dbl)  [unwired: 1 in, 1 out]
    n80 = local read "pequeoffset"() -> (w251:dbl)
    n81 = Multiply(x=w281, y=0.002713741718277) -> (x*y=w283:dbl)
    n82 = Multiply(x=w280, y=1.923167554010684) -> (x*y=w284:dbl)
    n83 = Multiply(x=w279, y=-0.925881295728961) -> (x*y=w282:dbl)
    n84 = local read "grandeoffset"() -> (w256:dbl)
    n85 = Select(t=w333, s="manual", f=w332) -> (s? t:f=w253:dbl)
    n86 = Compound Arithmetic op=ADD(w283, w284, w282) -> (w272:dbl)
    n87 = Select(t=w331, s="manual", f=w330) -> (s? t:f=w258:dbl)
    n88 = Add(x=w253, y=w251) -> (x+y=w252:dbl)
    n89 = Divide(x=-6498, y=6.283185307179586) -> (x/y=w363:dbl)
    n90 = Select(t=T1."Baja-abre", s="Garra", f=w297) -> (s? t:f=w300:T1)
    n91 = Add(x=w258, y=w256) -> (x+y=w257:dbl)
    n92 = Multiply(x=w363, y=w252) -> (x*y=w346:dbl)
    n93 = call <vilib>:"Read.vi"("error in (no error)"=w368, "Reset Counter"="Reset Counter", "Encoder Ref In"=w393) -> ("Counter Value"=w268:i32, "Encoder Ref Out"=w392:T12)  [unwired: 4 in, 3 out]
    n94 = Divide(x=-6534, y=6.283185307179586) -> (x/y=w360:dbl)
    n95 = Multiply(x=w360, y=w257) -> (x*y=w274:dbl)
    n96 = case shown="\"Baja-abre\"" w300 {
      tunnel: [T1."Up-Closed" w426 w435 w444] -> w298
      tunnel: [0.0 0.05 0.11 0.11] -> w289
      tunnel: [0.05 0.12 0.12 0.05] -> w288
      tunnel: w295 -> [_ _ w430 _]
      tunnel: [_ _ w429 _] -> w294
      tunnel: w293 -> [_ _ _ w440]
      tunnel: w292 -> [_ w422 _ _]
      tunnel: [_ w421 _ _] -> w291
      tunnel: [_ _ _ w439] -> w290
      frame "Up-Closed", Default {
      }
      frame "Baja-abre" {
        # "Hay que reiniciar contadores"
        n97 = Increment(x=w422) -> (x+1=w421:dbl)
        n98 = Less?(x=150.0, y=w421) -> (x < y?=w423:bool)
        n99 = Select(t=T1."cierra", s=w423, f=T1."Baja-abre") -> (s? t:f=w426:T1)
      }
      frame "cierra" {
        n100 = Increment(x=w430) -> (x+1=w429:dbl)
        n101 = Less?(x=150.0, y=w429) -> (x < y?=w433:bool)
        n102 = Select(t=T1."sube", s=w433, f=T1."cierra") -> (s? t:f=w435:T1)
      }
      frame "sube" {
        n103 = Increment(x=w440) -> (x+1=w439:dbl)
        n104 = Less?(x=150.0, y=w439) -> (x < y?=w441:bool)
        n105 = Select(t=T1."Up-Closed", s=w441, f=T1."sube") -> (s? t:f=w444:T1)
      }
    }
    n106 = xnode "PWM 2"("Duty Cycle"=w289, "Frequency [Hz]"=w370) -> ()  [unwired: 1 in, 1 out]
    n107 = xnode "PWM"("Duty Cycle"=w288, "Frequency [Hz]"=w370) -> ()  [unwired: 1 in, 1 out]
    n108 = Subtract(x=w268, y=w371) -> (x-y=w353:i32)
    n109 = Round To Nearest(number=w272) -> (nearest integer value=w396:dbl)
    n110 = Round To Nearest(number=w346) -> (nearest integer value=w391:dbl)
    n111 = call <vilib>:"Read.vi"("error in (no error)"=w369, "Reset Counter"="Reset Counter 2", "Encoder Ref In"=w407) -> ("Counter Value"=w269:i32, "Encoder Ref Out"=w402:T12)  [unwired: 4 in, 3 out]
    n112 = Subtract(x=w396, y=w269) -> (x-y=w260:dbl)
    n113 = Subtract(x=w391, y=w268) -> (x-y=w259:dbl)
    n114 = Multiply(x=w353, y=200) -> (x*y=w343:i32)
    n115 = Divide(x=6.283185307179586, y=6534) -> (x/y=w344:dbl)
    n116 = call "FiltroM2.vi"("Numeric 3"=w342, "Numeric in"=w341) -> ("Numeric out"=w340:dbl)  [unwired: 9 in]
    n117 = Multiply(x=w260, y=w344) -> (x*y=w270:dbl)
    n118 = Divide(x=6.283185307179586, y=6498) -> (x/y=w347:dbl)
    n119 = Multiply(x=w259, y=w347) -> (x*y=w310:dbl)
    n120 = Multiply(x=w347, y=w340) -> (x*y=w339:dbl)
    n121 = Divide(x=6.283185307179586, y=6498) -> (x/y=w336:dbl)
    n122 = Multiply(x=w336, y=w268) -> (x*y=w273:dbl)
    n123 = Multiply(x=w310, y=30.8878) -> (x*y=w372:dbl)
    n124 = Multiply(x=-2.3361, y=w339) -> (x*y=w345:dbl)
    n125 = Add(x=w372, y=w345) -> (x+y=w250:dbl)
    n126 = call "ObservadorPerturbacionPequeno.vi"("entrada planta"=w250, "salida planta"=w273, "xk +1"=w334) -> ("Perturbacion"=w301:dbl, "xk"=w335:T2)  [unwired: 7 in]
    n127 = feedback #1() -> (w277:bool)  [unwired: 1 in]
    n128 = call "PID2.vi"("Boolean"=w277, "Numeric in"=w270) -> ("Numeric out"=w249:dbl)  [unwired: 9 in]
    n129 = Multiply(x="saturacion", y=-1.0) -> (x*y=w357:dbl)
    n130 = Greater Or Equal?(x=w249, y="saturacion") -> (x >= y?=w398:bool)
    n131 = Less Or Equal?(x=w249, y=w357) -> (x <= y?=w397:bool)
    n132 = Multiply(x="saturacion 2", y=-1.0) -> (x*y=w264:dbl)
    n133 = shared-variable ".\\RT Variables.lvlib\\Homing"() -> (w384:bool)  [unwired: 1 in, 1 out]
    n134 = Or(x=w398, y=w397) -> (x .or. y?=w276:bool)
    n135 = feedback-in #1(w276) -> ()
    n136 = Greater Or Equal?(x=w250, y="saturacion 2") -> (x >= y?=w262:bool)
    n137 = Less Or Equal?(x=w250, y=w264) -> (x <= y?=w263:bool)
    n138 = case shown="False" w276 {
      tunnel: [w848 w850] -> w379
      tunnel: w249 -> [w849 _]
      frame False {
        n139 = Absolute Value(x=w849) -> (abs(x)=w848:dbl)
      }
      frame True {
        n140 = local read "saturacion"() -> (w850:dbl)
      }
    }
    n141 = Or(x=w262, y=w263) -> (x .or. y?=w267:bool)
    n142 = case shown="False" w267 {
      tunnel: [w414 w416] -> w261
      tunnel: w250 -> [w415 _]
      frame False {
        n143 = Absolute Value(x=w415) -> (abs(x)=w414:dbl)
      }
      frame True {
        n144 = local read "saturacion 2"() -> (w416:dbl)
      }
    }
    n145 = Select(t=T3."grande-Sensor" ("Enum"), s=w384, f=w381) -> (s? t:f=w349:T3)
    n146 = Get Date/Time In Seconds() -> (seconds since 1Jan1904=w413:timestamp)
    n147 = Bundle(w346, "Perturbacion"=w301, w273, "seconds since 1Jan1904"=w413, w274, w274, w270) -> (w275:T27)  [unwired: 1 in]
    n148 = xnode "Analog input (1 sample) 2"() -> ("sensor2 (A/AI2 (Pin 7))"=w366:dbl)  [unwired: 1 in, 1 out]
    "sensor2 (A/AI2 (Pin 7))" <- w366
    n149 = xnode "Analog input (1 sample)"() -> ("A/AI3 (Pin 9)"=w367:dbl)  [unwired: 1 in, 1 out]
    "sensor1" <- w367
    n150 = Greater?(x=w366, y=3.0) -> (0:w378:bool)
    n151 = Greater?(x=w367, y=3.0) -> (0:w380:bool)
    n152 = case shown="\"peque-sensor\"" w349 {
      tunnel: w261 -> [w532 _ _ _ _ w592]
      tunnel: [T3."normal" ("Enum") w547 w564 w575 w588 w594] -> w382
      tunnel: w380 -> [_ w542 _ _ _ _]
      tunnel: w379 -> [w534 w536 w549 w565 w576 w591]
      tunnel: [w534 w540 w554 w565 w576 w591] -> w271
      tunnel: w378 -> [_ _ _ w571 _ _]
      tunnel: [w532 0.0 ("f") 0.0 w569 w581 w592] -> w307
      tunnel: [_ _ w557 w572 _ w590] -> w376
      tunnel: [_ w542 w557 w572 _ w590] -> w374
      tunnel: [FALSE TRUE TRUE TRUE TRUE FALSE] -> w311
      tunnel: w260 -> [_ _ w556 _ _ _]
      tunnel: [0.0 w537 w550 _ _ _] -> w248
      tunnel: w259 -> [_ _ _ _ w580 _]
      tunnel: [0.0 1.0 1.0 _ _ _] -> w255
      tunnel: [_ _ _ 2.0 2.0 _] -> w254
      tunnel: [_ _ _ 1.0 -1.0 _] -> w247
      frame "normal", Default {
      }
      frame "grande-Sensor" {
        # "Planta"
        n153 = local write "saturacion"(0.35 ("f")) -> ()
        n154 = shared-variable ".\\RT Variables.lvlib\\Homing"(FALSE) -> ()  [unwired: 1 in, 1 out]
        n155 = Select(t=T3."grande home" ("Enum"), s=w542, f=T3."grande-Sensor" ("Enum")) -> (s? t:f=w547:T3)
        n156 = Absolute Value(x=w536) -> (abs(x)=w540:dbl)
        n157 = Multiply(x=w536, y=1.0) -> (x*y=w537:dbl)
      }
      frame "grande home" {
        w557 = FALSE
        # "Planta"
        n158 = Absolute Value(x=w556) -> (abs(x)=w561:dbl)
        n159 = local write "saturacion 2"(0.35) -> ()
        n160 = shared-variable ".\\RT Variables.lvlib\\Homing"(FALSE ("Homing")) -> ()  [unwired: 1 in, 1 out]
        n161 = Less?(x=w561, y=25.0) -> (x < y?=w552:bool)
        n162 = Select(t=T3."peque-sensor" ("Enum"), s=w552, f=T3."grande home" ("Enum")) -> (s? t:f=w564:T3)
        n163 = Absolute Value(x=w549) -> (abs(x)=w554:dbl)
        n164 = Multiply(x=w549, y=-1.0) -> (x*y=w550:dbl)
      }
      frame "peque-sensor" {
        w572 = TRUE
        # "sentido del pequeño esta en el grande"
        n165 = Select(t=T3."peque- home" ("Enum"), s=w571, f=T3."peque-sensor" ("Enum")) -> (s? t:f=w575:T3)
        n166 = Absolute Value(x=0.3 ("f")) -> (abs(x)=w569:dbl)
      }
      frame "peque- home" {
        n167 = Absolute Value(x=w580) -> (abs(x)=w585:dbl)
        n168 = Less?(x=w585, y=25.0) -> (x < y?=w583:bool)
        n169 = Select(t=T3."peque-reset" ("Enum"), s=w583, f=T3."peque- home" ("Enum")) -> (s? t:f=w588:T3)
        n170 = Absolute Value(x=-0.3 ("saturacion")) -> (abs(x)=w581:dbl)
      }
      frame "peque-reset" {
        w590 = TRUE
        n171 = Select(t=T3."normal" ("Enum"), s=w590, f=T3."peque-reset" ("Enum")) -> (s? t:f=w594:T3)
      }
    }
    n172 = Select(t=w248, s=w311, f=w249) -> (s? t:f=w312:dbl)
    n173 = Less Than 0?(x=w312) -> (x < 0?=w359:bool)
    n174 = Greater Or Equal To 0?(x=w312) -> (x >= 0?=w358:bool)
    n175 = xnode "Digital output (1 sample) 3"("A/DIO2 (Pin 15)"=w359) -> ()  [unwired: 1 in, 1 out]
    n176 = xnode "Digital output (1 sample) 4"("A/DIO3 (Pin 17)"=w358) -> ()  [unwired: 1 in, 1 out]
    n177 = local write "grandeoffset"(w255) -> ()
    n178 = local write "Reset Counter"(w376) -> ()
    n179 = local write "Reset Counter 2"(w374) -> ()
    n180 = local write "pequeoffset"(w254) -> ()
    n181 = Select(t=w247, s=w311, f=w250) -> (s? t:f=w348:dbl)
    n182 = xnode "Analog input (1 sample) 3"() -> ("stallBlanco (A/AI1 (Pin 5))"=w316:dbl, "stallRojo (A/AI0 (Pin 3))"=w318:dbl)  [unwired: 1 in, 1 out]
    "stallBlanco (A/AI1 (Pin 5))" <- w316
    "stallRojo (A/AI0 (Pin 3))" <- w318
    n183 = call <vilib>:"Set Duty Cycle.vi"("Duty Cycle"=w307, "PWM Ref In"=w383) -> ("error out"=w404:errorcluster, "PWM Ref Out"=w410:T5)  [unwired: 7 in]
    n184 = call <vilib>:"Set Duty Cycle.vi"("Duty Cycle"=w271, "PWM Ref In"=w406) -> ("error out"=w405:errorcluster, "PWM Ref Out"=w401:T5)  [unwired: 7 in]
    n185 = Multiply(x=0.987577800493881, y=w324) -> (x*y=w326:dbl)
    n186 = Multiply(x=0.012422199506119, y=w317) -> (x*y=w325:dbl)
    n187 = Multiply(x=0.987577800493881, y=w319) -> (x*y=w321:dbl)
    n188 = Multiply(x=0.012422199506119, y=w315) -> (x*y=w320:dbl)
    n189 = Add(x=w326, y=w325) -> (x+y=w314:dbl)
    n190 = Add(x=w321, y=w320) -> (x+y=w313:dbl)
    n191 = Merge Errors(w404, w405) -> (w403:errorcluster)
    n192 = shared-variable ".\\RT Variables.lvlib\\Stop RT Loops"() -> (w412:bool)  [unwired: 1 in, 1 out]
    n193 = Greater?(x=w314, y=0.1) -> (0:w386:bool)
    n194 = Greater?(x=w313, y=0.1) -> (0:w385:bool)
    n195 = shared-variable ".\\RT Variables.lvlib\\Data"(w275, error in=w403) -> (error out=w411:errorcluster)
    n196 = Or(x=w386, y=w385) -> (x .or. y?=w308:bool)
    n197 = Less Than 0?(x=w348) -> (x < 0?=w354:bool)
    n198 = Greater Or Equal To 0?(x=w348) -> (x >= 0?=w278:bool)
    n199 = Select(t=enum16{"No Stall", "Stall"}."Stall", s=w308, f=w303) -> (s? t:f=w306:enum16{"No Stall", "Stall"})
    n200 = Or(x=w411, y=w412) -> (x .or. y?=w400:bool)
    n201 = xnode "Digital output (1 sample)"("A/DIO0 (Pin 11)"=w354) -> ()  [unwired: 1 in, 1 out]
    n202 = xnode "Digital output (1 sample) 2"("A/DIO1 (Pin 13)"=w278) -> ()  [unwired: 1 in, 1 out]
    n203 = case shown="\"Stall\"" w306 {
      tunnel: [enum16{"No Stall", "Stall"}."No Stall" w451] -> w304
      tunnel: [FALSE ("stall") TRUE ("stall")] -> w302
      frame "No Stall", Default {
        # "aca quitaste lo de saturacion 0.7"
      }
      frame "Stall" {
        n204 = local write "saturacion"(0.0) -> ()
        n205 = feedback #2(0.0) -> (w458:dbl)
        n206 = Increment(x=w458) -> (x+1=w456:dbl)
        n207 = feedback-in #2(w456) -> ()
        n208 = Less?(x=1000.0, y=w456) -> (x < y?=w457:bool)
        n209 = Select(t=enum16{"No Stall", "Stall"}."No Stall", s=w457, f=enum16{"No Stall", "Stall"}."Stall") -> (s? t:f=w451:enum16{"No Stall", "Stall"})
      }
    }
    "stall" <- w302
    n210 = xnode "Button"() -> ("Value"=w309:bool)  [unwired: 1 in, 1 out]
    n211 = Or(x=w400, y=w309) -> (x .or. y?=w399:bool)
  }
  n212 = Destroy Stream Endpoint(8:w62, 11:w61) -> (0:w59:errorcluster)
  n213 = node-c288(w65) -> ()  [unwired: 1 out]
  n214 = case shown="Error" w54 {
    selector: w54 -> [w888 w889]
    tunnel: [w888 w889] -> w16
    frame No Error {
      # "No action required."
    }
    frame Error {
      # "Destroys Message network stream to stop Message loop, in case of error."
      n215 = shared-variable ".\\RT Variables.lvlib\\2setpoint"() -> (w890:refnum<k21>)  [unwired: 1 in, 1 out]
      n216 = Destroy Stream Endpoint(11:w890) -> ()  [unwired: 1 in, 1 out]
    }
  }
  n217 = call <vilib>:"Stop.vi"("error in (no error)"=w16, "Encoder Ref In"=w46) -> ("error out"=w47:errorcluster, "Encoder Ref Out"=w48:T12)  [unwired: 8 in]
  n218 = call <vilib>:"Stop.vi"("error in (no error)"=w16, "Encoder Ref In"=w15) -> ("error out"=w18:errorcluster, "Encoder Ref Out"=w19:T12)  [unwired: 8 in]
  n219 = call <vilib>:"Close.vi"("error in (no error)"=w47, "Encoder Ref In"=w48) -> ("error out"=w41:errorcluster)  [unwired: 9 in]
  n220 = call <vilib>:"Close.vi"("error in (no error)"=w18, "Encoder Ref In"=w19) -> ("error out"=w17:errorcluster)  [unwired: 9 in]
  n221 = call <vilib>:"Close.vi"("error in (no error)"=w41, "PWM Ref In"=w38) -> ("error out"=w40:errorcluster)  [unwired: 9 in]
  n222 = call <vilib>:"Close.vi"("error in (no error)"=w17, "PWM Ref In"=w14) -> ("error out"=w13:errorcluster)  [unwired: 9 in]
  n223 = Merge Errors(w59, w58, w40, w13) -> (w57:errorcluster)
  n224 = shared-variable "myRIO-1900\\Network Shared Variables.lvlib\\error IO"(w57) -> ()  [unwired: 1 in, 1 out]
